vi "DB - Count.vi"(5 "Include Inactive":bool=TRUE, 7 "subVI":bool=TRUE, 8 "error in (no error)":errorcluster, 10 "DB.dbo.Table":string="MyDB1.dbo.PartsDetails", 11 "Refnum in":T2) -> (0 "error out":errorcluster, 2 "COUNT":i32, 3 "Refnum out":T2)   [LabVIEW 2013]
uses:
  <vilib>/addons/database/Connection.llb/Conn ObjectReference.ctl
  <vilib>/addons/database/Connection.llb/Conn Execute.vi
  <vilib>/addons/database/Recordset.llb/Rec Fetch Recordset Data (R).vi
  <vilib>/addons/database/Recordset.llb/Rec Destroy - Connection.vi
  <vilib>/addons/database/Connection.llb/DB Tools Open Connec (String).vi
  <vilib>/addons/database/_DB Variant To Data/Database Variant To Data.xnode
  <vilib>/addons/database/NI_Database_API.lvlib
panel:
  out "call chain":string[](array[string])
  out "data":string[][](array[string])
  out "QUERY STRING":string
  out "COUNT":string
  in  "Connection Information":T1={"Connection "="SQL Server 32bit HPEnvy", "Username"="admin", "Password"="admin123"}
  # "Orders\nPartsDetails\nTransactions"
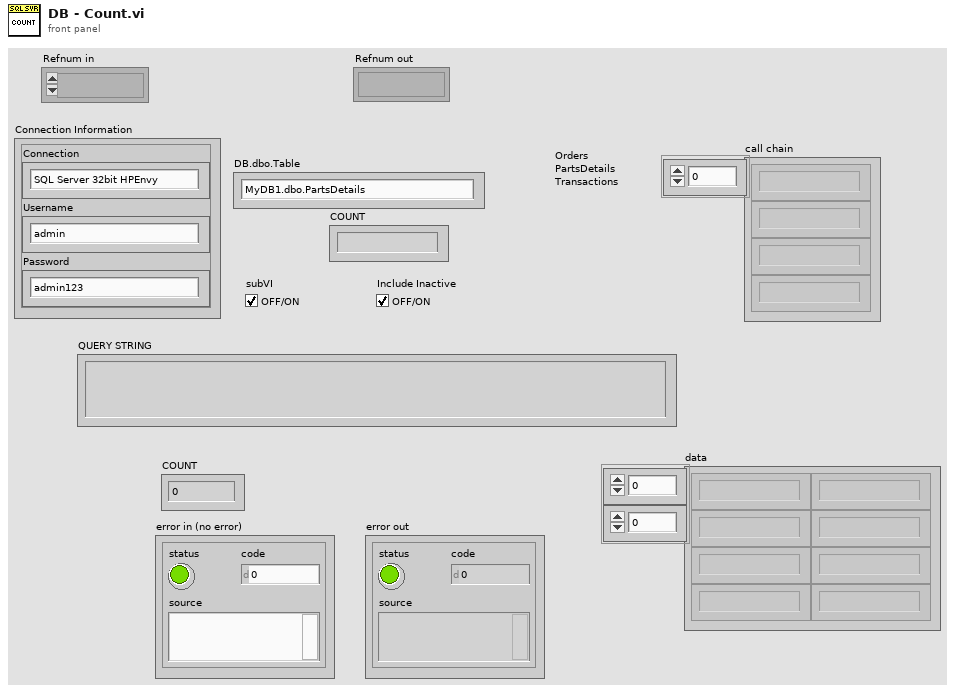
[diagram p1: front panel]
types:
  T1 = cluster{"Connection ":string, "Username":string, "Password":string}
  T2 = typedef "NI_Database_API.lvlib/Conn ObjectReference.ctl" = refnum<k1>
  T3 = typedef "DB - DB.Schema.Table.ctl" = cluster{"DB":string, "Schema":string, "Table":string}
  T4 = typedef "NI_Database_API.lvlib/Rec ObjectReference.ctl" = refnum<k1>
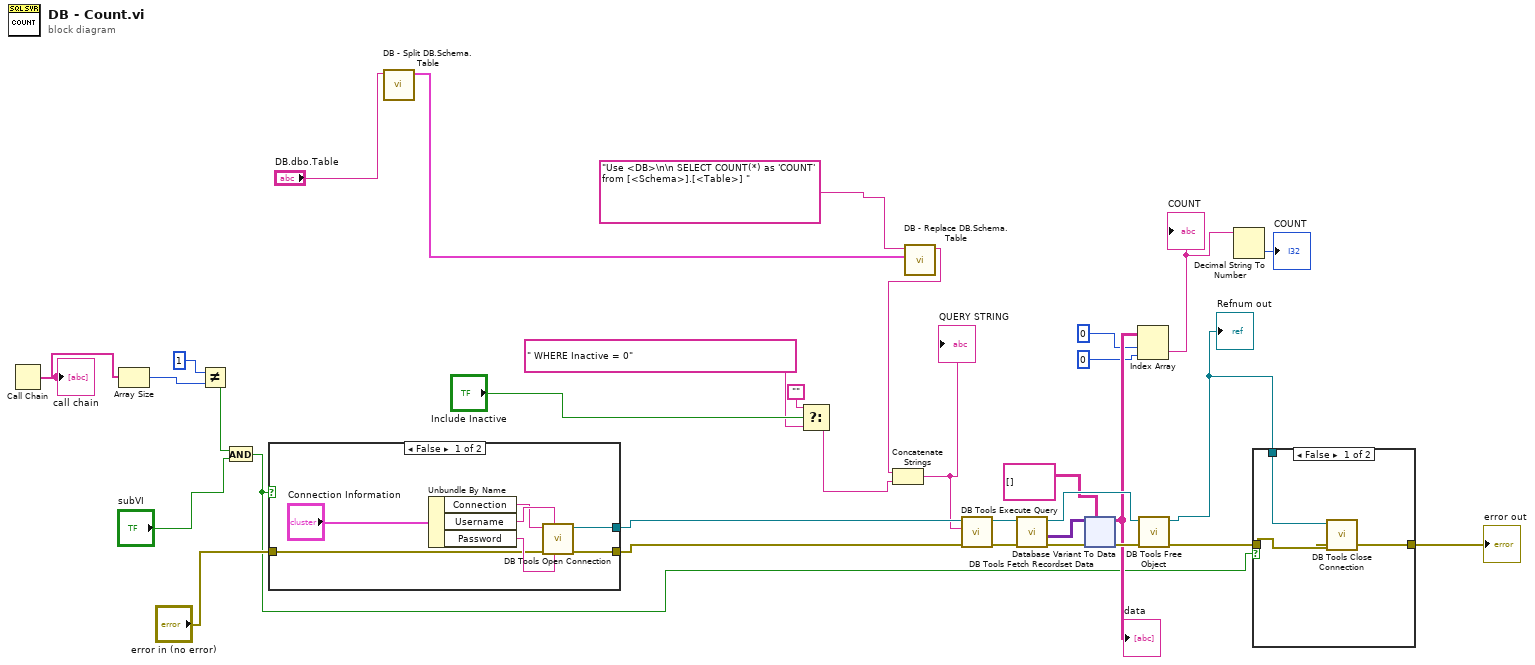
[diagram p0: block diagram]
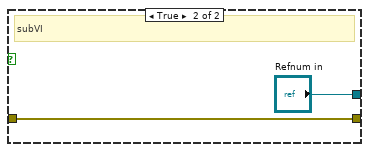
[diagram p3: hidden frame]
diagram:
  n1 = Call Chain() -> (call chain=w14:string[])
  "call chain" <- w14
  n2 = Array Size(array=w14) -> (size(s)=w13:i32)
  n3 = Not Equal?(x=1, y=w13) -> (x != y?=w12:bool)
  n4 = And(x=w12, y="subVI") -> (x .and. y?=w10:bool)
  n5 = case shown="False" w10 {
    tunnel: [w36 "Refnum in"] -> w25
    tunnel: "error in (no error)" -> [w35 w41]
    tunnel: [w34 w41] -> w26
    frame False {
      n6 = Unbundle By Name("Connection Information") -> ("Connection"=w38:string, "Username"=w39:string, "Password"=w37:string)
      n7 = call-poly <vilib>:"DB Tools Open Connection.vi"("password"=w37, "userID"=w39, "error in (no error)"=w35, "connection information"=w38) -> ("error out"=w34:errorcluster, "connection reference"=w36:T2)  [unwired: 4 in]
    }
    frame True {
      # "subVI"
    }
  }
  n8 = call "DB - Split DB.Schema.Table.vi"("DB.Schema.Table"="DB.dbo.Table") -> ("DB.Schema.Table"=w2:T3)  [unwired: 10 in]
  n9 = Select(t="", s="Include Inactive", f=" WHERE Inactive = 0" ("string")) -> (s? t:f=w6:string)
  n10 = call "DB - Replace DB.Schema.Table.vi"("DB.Schema.Table"=w2, "string in"="Use <DB>\n\n SELECT COUNT(*) as 'COUNT' from [<Schema>].[<Table>] " ("string")) -> ("string out"=w1:string)  [unwired: 8 in, 1 out]
  n11 = Concatenate Strings(w1, w6) -> (w21:string)
  "QUERY STRING" <- w21
  n12 = call-poly <vilib>:"DB Tools Execute Query.vi"("error in (no error)"=w26, "SQL query"=w21, "connection reference"=w25) -> ("error out"=w30:errorcluster, "recordset reference"=w28:T4)  [unwired: 5 in]
  n13 = call-poly <vilib>:"DB Tools Fetch Recordset Data.vi"("error in (no error)"=w30, "recordset reference"=w28) -> ("error out"=w32:errorcluster, "recordset data"=w31:variant[][], "recordset reference out"=w29:T4)  [unwired: 3 in]
  n14 = xnode "Database Variant To Data"("database variant"=w31, "error in (no error)"=w32, "type"=string[][] []) -> ("data"=w23:string[][], "error out"=w33:errorcluster)
  "data" <- w23
  n15 = Index Array(array=w23, index (row)=0 ("disabled index (row)"), index (col)=0) -> (element=w16:string)
  "COUNT" <- w16
  n16 = call-poly <vilib>:"DB Tools Free Object.vi"("error in (no error)"=w33, "recordset reference"=w29) -> ("error out"=w20:errorcluster, "connection reference"=w18:T2)  [unwired: 8 in]
  "Refnum out" <- w18
  n17 = Decimal String To Number(string=w16) -> (number=→"COUNT":i32)  [unwired: 2 in, 1 out]
  n18 = case shown="False" w10 {
    tunnel: w18 -> [w45 _]
    tunnel: w20 -> [w44 w46]
    tunnel: [w43 w46] -> w24
    frame False {
      n19 = call <vilib>:"DB Tools Close Connection.vi"("error in (no error)"=w44, "connection reference"=w45) -> ("error out"=w43:errorcluster)  [unwired: 5 in]
    }
    frame True {
      # "subVI"
    }
  }
  "error out" <- w24
